vi "Example_HVI_AOU-H0002.vi"() -> ()   [LabVIEW 2013]
uses:
  Instance           3 29Saved   Example_HVI_AOU-H0002 .vi
panel:
  out "VI Path":string
  in  "Frequency [Hz]":u64=10000000 max=200000000 step=1000000
  in  "Finish Program":bool
  in  "Amplitude [V]":dbl=0.5 min=-1.0 max=1.0 step=0.01 format="%#.4f"
  in  "Phase [degrees]":dbl min=0.0 max=360.0
  out "Get HVI-Module Status":errorcluster
  out "HVI open Status":errorcluster
  in  "Module name in HVI":string="AOU"
  out "Close HVI Status":errorcluster
  in  "HVI file":string="Example_HVI_AOU.HVI"
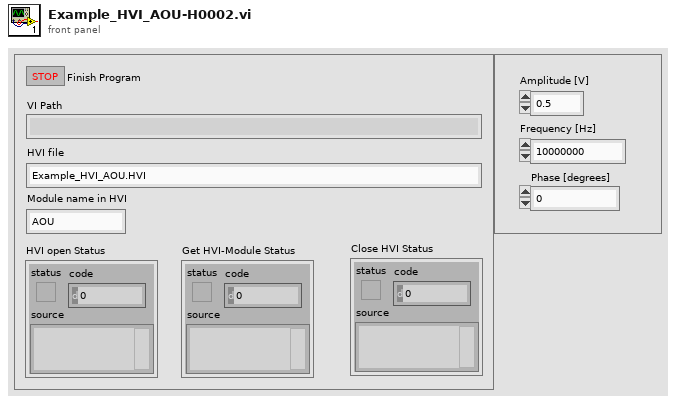
[diagram p1: front panel]
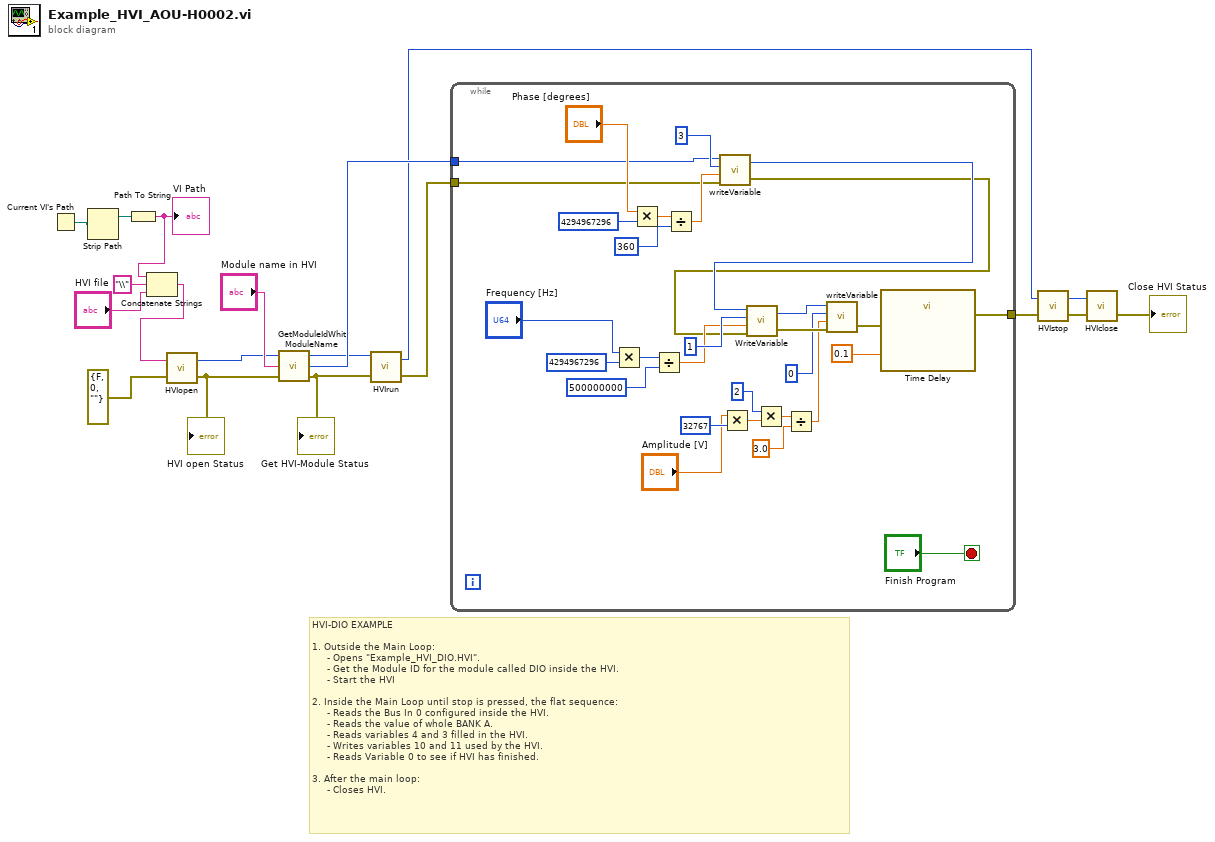
[diagram p0: block diagram]
diagram:
  # "HVI-DIO EXAMPLE\n\n1. Outside the Main Loop:\n     - Opens \"Example_HVI_DIO.HVI\".\n     - Get the Module ID for the module called DIO inside the HVI.\n     - Start the HVI\n\n2. Inside the Main Loop until stop is pressed, the flat sequence:\n     - Reads the Bus In 0 configured inside the HVI.\n     - Reads the value of whole BANK A.\n     - Reads variables 4 and 3 filled in the HVI.\n     - Writes variables 10 and 11 used by the HVI.\n     - Reads Variable 0 to see if HVI has finished.\n\n3. After the main loop:\n     - Closes HVI."
  n1 = Current VI's Path() -> (path=w11:path)
  n2 = Strip Path(path=w11) -> (stripped path=w10:path)  [unwired: 1 out]
  n3 = Path To String(path=w10) -> (string=w9:string)
  "VI Path" <- w9
  n4 = Concatenate Strings(w9, "\\" ("string"), "HVI file") -> (w7:string)
  n5 = call <vilib>:"HVIopen.vi"("errorIn"=errorcluster {"status"=FALSE, "code"=0, "source"=""}, "HVIfile"=w7) -> ("errorOut"=w5:errorcluster, "HVIID"=w4:i32)
  "HVI open Status" <- w5
  n6 = call <vilib>:"GetModuleIdWhitModuleName.vi"("errorIn"=w5, "ModuleName"="Module name in HVI", "HVIID"=w4) -> ("errorOut"=w16:errorcluster, "ModuleID"=w18:u32, "HVIIDOut"=w17:i32)
  "Get HVI-Module Status" <- w16
  n7 = call <vilib>:"HVIrun.vi"("errorIn"=w16, "HVIID"=w17) -> ("errorOut"=w15:errorcluster, "HVIIDOut"=w13:i32)
  n8 = while {
    tunnel: w18 -> [w28]
    tunnel: w15 -> [w27]
    tunnel: [w46] -> w14
    stop <- "Finish Program" stop-if-true
    n9 = Multiply(x="Frequency [Hz]", y=i64 4294967296) -> (x*y=w37:u64)
    n10 = Multiply(x="Phase [degrees]", y=i64 4294967296) -> (x*y=w32:dbl)
    n11 = Divide(x=w37, y=u64 500000000) -> (x/y=w39:dbl)
    n12 = Divide(x=w32, y=u64 360) -> (x/y=w30:dbl)
    n13 = call <vilib>:"writeVariable.vi"("errorIn"=w27, "Value"=w30, "Number"=3, "ModuleID"=w28) -> ("errorOut"=w25:errorcluster, "ModuleIDOut"=w26:i32)
    n14 = Multiply(x="Amplitude [V]", y=u64 32767) -> (x*y=w24:dbl)
    n15 = call <vilib>:"WriteVariable.vi"("errorIn"=w25, "Value"=w39, "Number"=1 ("Number variable\nHVI runinng 3"), "ModuleID"=w26) -> ("errorOut"=w44:errorcluster, "ModuleIDOut"=w43:i32)
    n16 = Multiply(x=u64 2 ("y"), y=w24) -> (x*y=w22:dbl)
    n17 = Divide(x=w22, y=3.0) -> (x/y=w21:dbl)
    n18 = call <vilib>:"writeVariable.vi"("errorIn"=w44, "Value"=w21, "Number"=0, "ModuleID"=w43) -> ("errorOut"=w47:errorcluster)  [unwired: 1 out]
    n19 = call "Time Delay"("error in (no error)"=w47, "Delay Time (s)"=0.1) -> ("error out"=w46:errorcluster)  [unwired: 9 in]
  }
  n20 = call <vilib>:"HVIstop.vi"("errorIn"=w14, "HVIID"=w13) -> ("errorOut"=w2:errorcluster, "HVIIDOut"=w1:i32)
  n21 = call <vilib>:"HVIclose.vi"("errorIn"=w2, "HVIID"=w1) -> ("errorOut"=→"Close HVI Status":errorcluster)  [unwired: 1 in]
